vi "SetSpeed.vi"(8 "error in (no error)":errorcluster, 10 "Speed":i32, 11 "Motor in":refnum<class "Motor.lvclass">) -> (0 "error out":errorcluster, 3 "Motor out":refnum<class "Motor.lvclass">)   [LabVIEW 2019, in "Motor.lvclass"]
uses:
  Motor.lvclass
  Motor.lvclass/Motor.ctl
  Motor Serial class/Serial.lvclass
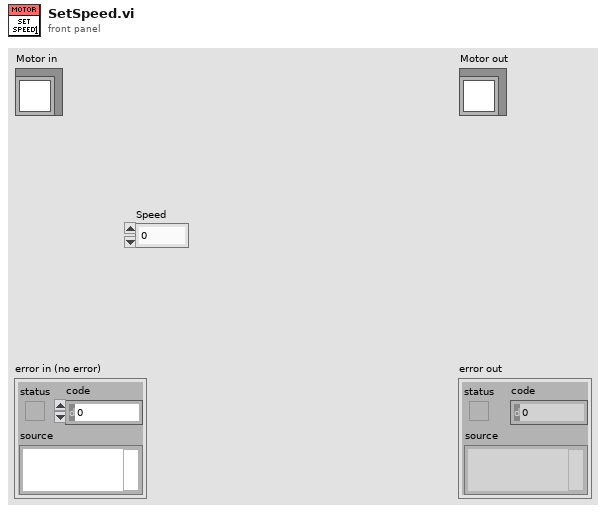
[diagram p1: front panel]
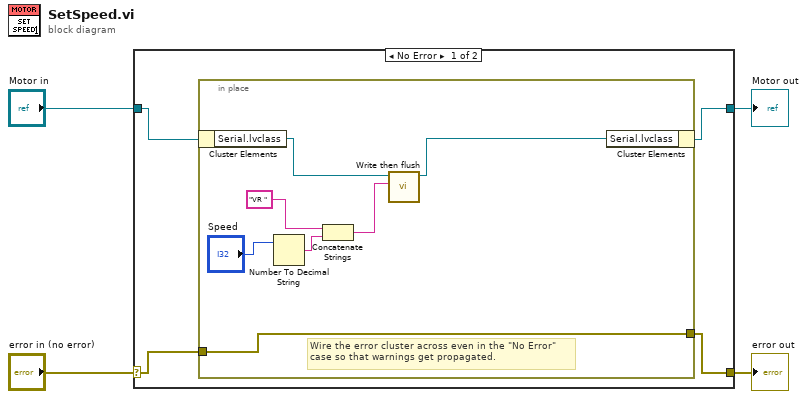
[diagram p0: block diagram]
diagram:
  n1 = case shown="No Error" "error in (no error)" {
    selector: "error in (no error)" -> [w6 w17]
    tunnel: [w5 w17] -> w3
    tunnel: [w7 w16] -> w1
    tunnel: "Motor in" -> [w8 w16]
    frame No Error {
      n2 = in-place {
        in-place-border: w6 -> [w15]
        in-place-border: [w15] -> w5
        # "Wire the error cluster across even in the \"No Error\"\ncase so that warnings get propagated."
        n3 = in-place-cluster #1(w8) -> ("Serial.lvclass"=w14:refnum<class "Serial.lvclass">)
        n4 = Number To Decimal String(number="Speed") -> (decimal integer string=w10:string)  [unwired: 1 in]
        n5 = Concatenate Strings("VR " ("string"), w10) -> (w11:string)
        n6 = call "Write then flush.vi"("TX Data"=w11, "Motor_Serial in"=w14) -> ("Motor_Serial out"=w13:refnum<class "Serial.lvclass">)  [unwired: 8 in, 1 out]
        n7 = in-place-cluster #1("Serial.lvclass"=w13) -> (w7:refnum<class "Motor.lvclass">)
      }
    }
    frame Error {
    }
  }
  "error out" <- w3
  "Motor out" <- w1
